vi "rsscope_FormatSearchNameSourceReal64_WriteCallback.vi"(5 "Attribute":T1={"Identifier"="", "Descriptive Name"="", "Data Type"=enum."Integer 32", "Command"="", "Access"=enum."Read/Write", "Range Table"="", "Read Callback"="", "Write Callback"="", "Supported Models"="", "Instrument Options"="", "Index"=0, "OPC Wait"=FALSE, "No Status Check"=FALSE, "Cache Only"=FALSE}, 7 "Repeated Capability":string, 8 "error in (no error)":errorcluster, 10 "Attribute Value Double":dbl, 11 "VISA resource name":refnum<visa-resource-name>) -> (0 "error out":errorcluster, 3 "VISA resource name out":refnum<visa-resource-name>)   [LabVIEW 2018]
doc: "This VI sets the attribute value.\n\nThis is a low-level VI that you can use to set the values of instrument-specific properties and inherent IVI properties. If the property represents an instrument state, this VI performs instrument I/O in the following cases:\n\n- State caching is disabled for the entire session or for the particular property.\n\n- State caching is enabled and the currently cached value is invalid or is different than the value you specify. \n\nThis instrument driver contains high-level VIs that set most of the instrument properties. It is best to use the high-level driver VIs as much as possible. They handle order dependencies and multithread locking for you. In addition, they perform status checking only after setting all of the properties. In contrast, when you set multiple properties using the SetAttribute VIs, the VIs check the instrument status after each call.\n\nAlso, when state caching is enabled, the high-level VIs that configure multiple properties perform instrument I/O only for the properties whose value you change. Thus, you can safely call the high-level VIs without the penalty of redundant instrument I/O."
uses:
  rsidr_core.llb/type_Attribute.ctl
  rsidr_core.llb/type_Attribute_Data_Type.ctl
  rsidr_core.llb/type_ReadWriteAccess.ctl
  rsidr_core.llb/rsscope_rsidr_core.lvlib
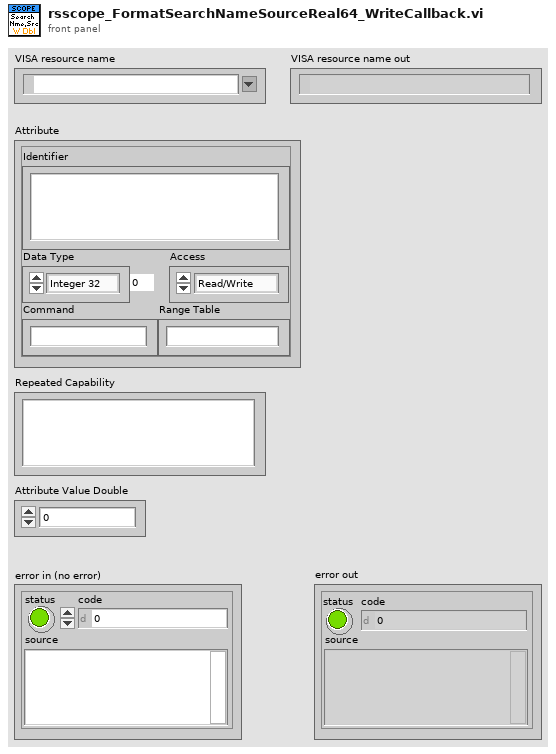
[diagram p1: front panel]
types:
  T1 = typedef "rsscope_rsidr_core.lvlib/type_Attribute.ctl" = cluster{"Identifier":string, "Descriptive Name":string, "Data Type":T2, "Command":string, "Access":T3, "Range Table":string, "Read Callback":string, "Write Callback":string, "Supported Models":string, "Instrument Options":string, "Index":i32, "OPC Wait":bool, "No Status Check":bool, "Cache Only":bool}
  T2 = typedef "rsscope_rsidr_core.lvlib/type_Attribute_Data_Type.ctl" = enum16{"Integer 32", "Double", "String", "Boolean", "None", "Integer 64", "RawString"}
  T3 = typedef "rsscope_rsidr_core.lvlib/type_ReadWriteAccess.ctl" = enum16{"Read Only", "Write Only", "Read/Write"}
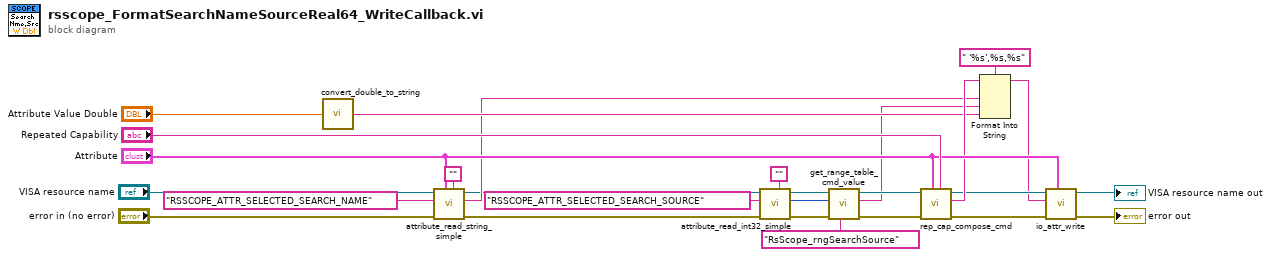
[diagram p0: block diagram]
diagram:
  n1 = call "convert_double_to_string.vi"("double in"="Attribute Value Double") -> ("string out"=w13:string)  [unwired: 4 in]
  n2 = call "attribute_read_string_simple.vi"("Repeated Capability"="" ("Empty String Constant"), "Attribute"="Attribute", "error in"="error in (no error)", "Direct Attribute ID (\"\")"="RSSCOPE_ATTR_SELECTED_SEARCH_NAME" ("Direct Attribute ID (\"\")"), "VISA resource name"="VISA resource name") -> ("error out"=w8:errorcluster, "String out"=w12:string, "VISA resource name out"=w7:refnum<visa-resource-name>)  [unwired: 4 in]
  n3 = call "attribute_read_int32_simple.vi"("Repeated Capability"="" ("Empty String Constant"), "error in"=w8, "Direct Attribute ID (\"\")"="RSSCOPE_ATTR_SELECTED_SEARCH_SOURCE" ("Direct Attribute ID (\"\")"), "VISA resource name"=w7) -> ("error out"=w6:errorcluster, "Int32 out"=w10:i32, "VISA resource name out"=w5:refnum<visa-resource-name>)  [unwired: 5 in]
  n4 = call "get_range_table_cmd_value.vi"("Range Table ID in"="RsScope_rngSearchSource", "error in"=w6, "Input Int32 value"=w10, "VISA resource name"=w5) -> ("error out"=w4:errorcluster, "Cmd value out"=w1:string, "VISA resource name out"=w3:refnum<visa-resource-name>)  [unwired: 5 in]
  n5 = call "rep_cap_compose_cmd.vi"("Repeated Capability"="Repeated Capability", "Attribute"="Attribute", "error in"=w4, "VISA resource name"=w3) -> ("error out"=w16:errorcluster, "Command out"=w18:string, "VISA resource name out"=w17:refnum<visa-resource-name>)  [unwired: 5 in]
  n6 = Format Into String(format string=" '%s',%s,%s", initial string=w18, w12, w1, w13) -> (resulting string=w15:string)  [unwired: 1 in, 1 out]
  n7 = call "io_attr_write.vi"("Attribute"="Attribute", "error in"=w16, "write buffer"=w15, "VISA resource name"=w17) -> ("error out"=→"error out":errorcluster, "VISA resource name out"=→"VISA resource name out":refnum<visa-resource-name>)  [unwired: 6 in]
